vi "Unflatten LIDAR Data.vi"(0 "LIDAR Data":cluster{"Magnitude":dbl[], "Direction":dbl[]}) -> (4 "Range (m)":dbl[](array[numeric]), 6 "Bearing (rad)":dbl[](array[numeric]))   [LabVIEW 2012]
uses:
  Utilities/Robot Parameters/Robot Parameters.vi
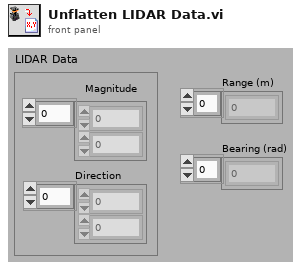
[diagram p1: front panel]
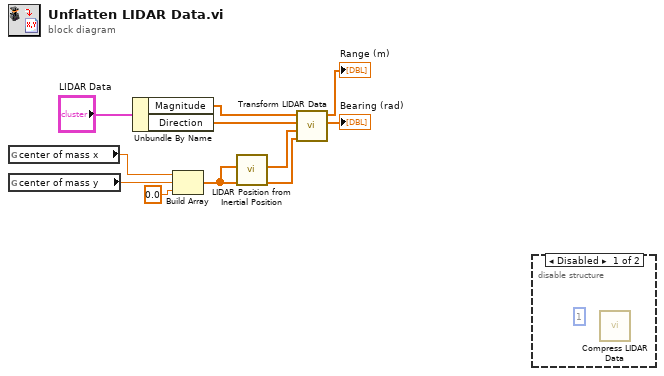
[diagram p0: block diagram]
diagram:
  n1 = global read "Robot Parameters.vi" "center of mass x"() -> (w5:dbl)
  n2 = global read "Robot Parameters.vi" "center of mass y"() -> (w4:dbl)
  n3 = Unbundle By Name("LIDAR Data") -> ("Magnitude"=w2:dbl[], "Direction"=w1:dbl[])
  n4 = Build Array(w5, w4, 0.0 ("center of mass y")) -> (w6:dbl[])
  n5 = call "LIDAR Position from Inertial Position.vi"("CM X, Y, Theta"=w6) -> ("LIDAR X, Y, Theta"=w10:dbl[])  [unwired: 10 in]
  n6 = call "Transform LIDAR Data.vi"("New Orientation (X m, Y m, T rad)"=w6, "Orientation (X m, Y m, T rad)"=w10, "Direction (deg)"=w1, "Magnitude (mm)"=w2) -> ("Direction out (rad)"=→"Bearing (rad)":dbl[], "Magnitude out (m)"=→"Range (m)":dbl[])  [unwired: 5 in, 1 out]
  n7 = disable-structure shown="Disabled" {
    frame Disabled {
      (unwired) 1 ("compress")
      n8 = call "Compress LIDAR Data.vi"() -> ()  [unwired: 10 in, 2 out]
    }
    frame Enabled {
    }
  }
